vi "XAIOSCBG_v1.VI"(0 "BoardNum":u32, 1 "signal type":T2(ring)=enum."Sawtooth" caption="Signal Type", 2 "LowChan":i32, 3 "HighChan":i32=1, 5 "number of points":dbl=1024.0, 7 "amplitude (1.0)":dbl=10.0 caption="Amplitude (Volts)", 9 "offset (0.0)":dbl caption="Offset (Volts)", 11 "Range":i32(ring)=1 items=["Not Programmable"=0, "+- 20 V"=27, "+- 10 V"=1, "+- 5 V"=2, "+- 4 V"=28, "+- 2.5 V"=3, "+- 2 V"=29, "+- 1.67 V"=4, "+- 1.25 V"=5, "+- 1 V"=6, "+- .625 V"=7, "+- .5 V"=8, "+- .25 V"=30, "+- .2 V"=31, "+- .1 V"=9, "+- .05 V"=10, "+- .01 V"=11, "+- .005 V"=12, "0 - 10 V"=13, "0 - 5 V"=14, "0 - 4 V"=36, "0 - 2.5 V"=15, "0 - 2 V"=16, "0 - 1.67 V"=17, "0 - 1.25 V"=18, "0 - 1 V"=19, "0 - .5 V"=32, "0 - .25 V"=33, "0 - .2 V"=34, "0 - .1 V"=20, "0 - .02 V"=35, "0 - .01 V"=21, "4 - 20 mA"=22, "2 - 10 mA"=23, "1 - 5 mA"=24, ".5 - 2.5 mA"=25, "0 - 20 mA"=26], 12 "Rate":dbl=100.0, 13 "HighAOChan":i32, 14 "LowAOChan":i32) -> (4 "Output Array":dbl[][](array[numeric])=[[0.0, 0.006135884649154475, 0.012271538285719925, 0.01840672990580482, 0.024541228522912288, 0.030674803176636626, 0.03680722294135883, 0.04293825693494082, 0.049067674327418015, 0.05519524434968994, 0.06132073630220858, 0.06744391956366406, 0.07356456359966743, 0.07968243797143013, 0.0857973123444399, 0.09190895649713272, 0.0980171403295606, 0.10412163387205457, 0.11022220729388306, 0.11631863091190477, 0.1224106751992162, 0.12849811079379317, 0.1345807085071262, 0.14065823933284924, 0.14673047445536175, 0.15279718525844344, 0.15885814333386145, 0.16491312048996992, 0.17096188876030122, 0.17700422041214875, 0.18303988795514095, 0.18906866414980622, 0.19509032201612828, 0.2011046348420919, 0.20711137619221856, 0.21311031991609136, 0.2191012401568698, 0.22508391135979283, 0.2310581082806711, 0.2370236059943672, 0.2429801799032639, 0.24892760574572018, 0.25486565960451457, 0.2607941179152755, 0.26671275747489837, 0.272621355449949, 0.2785196893850531, 0.2844075372112718, 0.2902846772544624, 0.29615088824362384, 0.3020059493192281, 0.30784964004153487, 0.31368174039889146, 0.3195020308160157, 0.3253102921622629, 0.33110630575987643, 0.33688985339222005, 0.3426607173119944, 0.34841868024943456, 0.3541635254204904, 0.35989503653498817, 0.36561299780477385, 0.37131719395183754, 0.37700741021641826, 0.3826834323650898, 0.3883450466988263, 0.3939920400610481, 0.39962419984564684, 0.40524131400498986, 0.41084317105790397, 0.4164295600976372, 0.4220002707997997, 0.4275550934302821, 0.43309381885315196, 0.43861623853852766, 0.44412214457042926, 0.4496113296546066, 0.45508358712634384, 0.46053871095824, 0.4659764957679662, 0.47139673682599764, 0.47679923006332214, 0.4821837720791228, 0.48755016014843594, 0.49289819222978404, 0.49822766697278187, 0.5035383837257176, 0.508830142543107, 0.5141027441932218, 0.5193559901655896, 0.524589682678469, 0.5298036246862947, 0.5349976198870973, 0.5401714727298929, 0.5453249884220465, 0.5504579729366048, 0.5555702330196022, 0.560661576197336, 0.5657318107836132, 0.5707807458869673, 0.5758081914178453, 0.5808139580957645, 0.5857978574564389, 0.5907597018588743, 0.5956993044924334, 0.600616479383869, 0.6055110414043255, 0.6103828062763095, 0.6152315905806268, 0.6200572117632892, 0.6248594881423863, 0.629638238914927, 0.6343932841636455, 0.6391244448637757, 0.6438315428897915, 0.6485144010221124, 0.6531728429537768, 0.6578066932970786, 0.6624157775901718, 0.6669999223036375, 0.6715589548470184, 0.6760927035753159, 0.680600997795453, 0.6850836677727004, 0.6895405447370669, 0.693971460889654, 0.6983762494089728, 0.7027547444572253, 0.7071067811865476, 0.7114321957452164, 0.7157308252838187, 0.7200025079613817, 0.7242470829514669, 0.7284643904482252, 0.7326542716724128, 0.7368165688773699, 0.7409511253549591, 0.745057785441466, 0.7491363945234594, 0.7531867990436125, 0.7572088465064846, 0.7612023854842618, 0.765167265622459, 0.7691033376455796, 0.773010453362737, 0.7768884656732324, 0.7807372285720945, 0.7845565971555752, 0.7883464276266062, 0.7921065773002124, 0.7958369046088836, 0.799537269107905, 0.8032075314806449, 0.8068475535437992, 0.8104571982525948, 0.8140363297059484, 0.8175848131515837, 0.8211025149911046, 0.8245893027850253, 0.8280450452577558, 0.8314696123025452, 0.83486287498638, 0.8382247055548381, 0.8415549774368984, 0.8448535652497071, 0.8481203448032972, 0.8513551931052652, 0.8545579883654005, 0.8577286100002721, 0.8608669386377673, 0.8639728561215867, 0.8670462455156926, 0.8700869911087115, 0.8730949784182901, 0.8760700941954066, 0.8790122264286335, 0.881921264348355, 0.8847970984309378, 0.8876396204028539, 0.8904487232447579, 0.8932243011955153, 0.8959662497561851, 0.8986744656939538, 0.901348847046022, 0.9039892931234433, 0.9065957045149153, 0.9091679830905224, 0.9117060320054299, 0.9142097557035307, 0.9166790599210427, 0.9191138516900578, 0.9215140393420419, 0.9238795325112867, 0.9262102421383114, 0.9285060804732156, 0.9307669610789837, 0.9329927988347388, 0.9351835099389476, 0.937339011912575, 0.9394592236021899, 0.9415440651830208, 0.9435934581619604, 0.9456073253805213, 0.9475855910177411, 0.9495281805930367, 0.9514350209690083, 0.9533060403541939, 0.9551411683057707, 0.9569403357322088, 0.9587034748958716, 0.9604305194155658, 0.9621214042690416, 0.9637760657954398, 0.9653944416976894, 0.9669764710448521, 0.9685220942744173, 0.970031253194544, 0.9715038909862518, 0.9729399522055602, 0.9743393827855759, 0.9757021300385286, 0.9770281426577544, 0.9783173707196277, 0.9795697656854405, 0.9807852804032304, 0.9819638691095552, 0.9831054874312163, 0.984210092386929, 0.9852776423889412, 0.9863080972445987, 0.9873014181578584, 0.9882575677307495, 0.989176509964781, 0.9900582102622971, 0.99090263542778, 0.9917097536690995, 0.99247953459871, 0.9932119492347945, 0.9939069700023561, 0.9945645707342554, 0.9951847266721969, 0.9957674144676598, 0.996312612182778, 0.9968202992911657, 0.9972904566786902, 0.9977230666441916, 0.9981181129001492, 0.9984755805732948, 0.9987954562051724, 0.9990777277526454, 0.9993223845883495, 0.9995294175010931, 0.9996988186962042, 0.9998305817958234, 0.9999247018391445, 0.9999811752826011, 1.0, 0.9999811752826011, 0.9999247018391445, 0.9998305817958234, 0.9996988186962042, 0.9995294175010931, 0.9993223845883495, 0.9990777277526454, 0.9987954562051724, 0.9984755805732948, 0.9981181129001492, 0.9977230666441916, 0.9972904566786902, 0.9968202992911657, 0.996312612182778, 0.9957674144676598, 0.9951847266721969, 0.9945645707342554, 0.9939069700023561, 0.9932119492347945, 0.99247953459871, 0.9917097536690995, 0.99090263542778, 0.9900582102622971, 0.989176509964781, 0.9882575677307495, 0.9873014181578584, 0.9863080972445987, 0.9852776423889412, 0.984210092386929, 0.9831054874312163, 0.9819638691095552, 0.9807852804032304, 0.9795697656854405, 0.9783173707196277, 0.9770281426577544, 0.9757021300385286, 0.9743393827855759, 0.9729399522055602, 0.9715038909862518, 0.970031253194544, 0.9685220942744173, 0.9669764710448521, 0.9653944416976894, 0.9637760657954398, 0.9621214042690416, 0.9604305194155658, 0.9587034748958716, 0.9569403357322088, 0.9551411683057707, 0.9533060403541939, 0.9514350209690083, 0.9495281805930367, 0.9475855910177411, 0.9456073253805213, 0.9435934581619604, 0.9415440651830208, 0.9394592236021899, 0.937339011912575, 0.9351835099389476, 0.9329927988347388, 0.9307669610789837, 0.9285060804732156, 0.9262102421383114, 0.9238795325112867, 0.9215140393420419, 0.9191138516900578, 0.9166790599210427, 0.9142097557035307, 0.9117060320054299, 0.9091679830905224, 0.9065957045149153, 0.9039892931234433, 0.901348847046022, 0.8986744656939538, 0.8959662497561851, 0.8932243011955153, 0.8904487232447579, 0.8876396204028539, 0.8847970984309378, 0.881921264348355, 0.8790122264286335, 0.8760700941954066, 0.8730949784182901, 0.8700869911087115, 0.8670462455156926, 0.8639728561215867, 0.8608669386377673, 0.8577286100002721, 0.8545579883654005, 0.8513551931052652, 0.8481203448032972, 0.8448535652497071, 0.8415549774368984, 0.8382247055548381, 0.83486287498638, 0.8314696123025452, 0.8280450452577558, 0.8245893027850253, 0.8211025149911046, 0.8175848131515837, 0.8140363297059484, 0.8104571982525948, 0.8068475535437992, 0.8032075314806449, 0.799537269107905, 0.7958369046088836, 0.7921065773002124, 0.7883464276266062, 0.7845565971555752, 0.7807372285720945, 0.7768884656732324, 0.773010453362737, 0.7691033376455796, 0.765167265622459, 0.7612023854842618, 0.7572088465064846, 0.7531867990436125, 0.7491363945234594, 0.745057785441466, 0.7409511253549591, 0.7368165688773699, 0.7326542716724128, 0.7284643904482252, 0.7242470829514669, 0.7200025079613817, 0.7157308252838187, 0.7114321957452164, 0.7071067811865476, 0.7027547444572253, 0.6983762494089728, 0.693971460889654, 0.6895405447370669, 0.6850836677727004, 0.680600997795453, 0.6760927035753159, 0.6715589548470184, 0.6669999223036375, 0.6624157775901718, 0.6578066932970786, 0.6531728429537768, 0.6485144010221124, 0.6438315428897915, 0.6391244448637757, 0.6343932841636455, 0.629638238914927, 0.6248594881423863, 0.6200572117632892, 0.6152315905806268, 0.6103828062763095, 0.6055110414043255, 0.600616479383869, 0.5956993044924334, 0.5907597018588743, 0.5857978574564389, 0.5808139580957645, 0.5758081914178453, 0.5707807458869673, 0.5657318107836132, 0.560661576197336, 0.5555702330196022, 0.5504579729366048, 0.5453249884220465, 0.5401714727298929, 0.5349976198870973, 0.5298036246862947, 0.524589682678469, 0.5193559901655896, 0.5141027441932218, 0.508830142543107, 0.5035383837257176, 0.49822766697278187, 0.49289819222978404, 0.48755016014843594, 0.4821837720791228, 0.47679923006332214, 0.47139673682599764, 0.4659764957679662, 0.46053871095824, 0.45508358712634384, 0.4496113296546066, 0.44412214457042926, 0.43861623853852766, 0.43309381885315196, 0.4275550934302821, 0.4220002707997997, 0.4164295600976372, 0.41084317105790397, 0.40524131400498986, 0.39962419984564684, 0.3939920400610481, 0.3883450466988263, 0.3826834323650898, 0.37700741021641826, 0.37131719395183754, 0.36561299780477385, 0.35989503653498817, 0.3541635254204904, 0.34841868024943456, 0.3426607173119944, 0.33688985339222005, 0.33110630575987643, 0.3253102921622629, 0.3195020308160157, 0.31368174039889146, 0.30784964004153487, 0.3020059493192281, 0.29615088824362384, 0.2902846772544624, 0.2844075372112718, 0.2785196893850531, 0.272621355449949, 0.26671275747489837, 0.2607941179152755, 0.25486565960451457, 0.24892760574572018, 0.2429801799032639, 0.2370236059943672, 0.2310581082806711, 0.22508391135979283, 0.2191012401568698, 0.21311031991609136, 0.20711137619221856, 0.2011046348420919, 0.19509032201612828, 0.18906866414980622, 0.18303988795514095, 0.17700422041214875, 0.17096188876030122, 0.16491312048996992, 0.15885814333386145, 0.15279718525844344, 0.14673047445536175, 0.14065823933284924, 0.1345807085071262, 0.12849811079379317, 0.1224106751992162, 0.11631863091190477, 0.11022220729388306, 0.10412163387205457, 0.0980171403295606, 0.09190895649713272, 0.0857973123444399, 0.07968243797143013, 0.07356456359966743, 0.06744391956366405, 0.06132073630220858, 0.05519524434968994, 0.049067674327418015, 0.04293825693494082, 0.03680722294135883, 0.030674803176636626, 0.024541228522912288, 0.01840672990580482, 0.012271538285719925, 0.006135884649154475, -5.421010862427522e-20, -0.006135884649154475, -0.012271538285719925, -0.01840672990580482, -0.024541228522912288, -0.030674803176636626, -0.03680722294135883, -0.04293825693494082, -0.049067674327418015, -0.05519524434968994, -0.06132073630220858, -0.06744391956366406, -0.07356456359966743, -0.07968243797143013, -0.0857973123444399, -0.09190895649713272, -0.0980171403295606, -0.10412163387205457, -0.11022220729388306, -0.11631863091190477, -0.1224106751992162, -0.12849811079379317, -0.1345807085071262, -0.14065823933284924, -0.14673047445536175, -0.15279718525844344, -0.15885814333386145, -0.16491312048996992, -0.17096188876030122, -0.17700422041214875, -0.18303988795514095, -0.18906866414980622, -0.19509032201612828, -0.2011046348420919, -0.20711137619221856, -0.21311031991609136, -0.2191012401568698, -0.22508391135979283, -0.2310581082806711, -0.2370236059943672, -0.2429801799032639, -0.24892760574572018, -0.25486565960451457, -0.2607941179152755, -0.26671275747489837, -0.272621355449949, -0.2785196893850531, -0.2844075372112718, -0.2902846772544624, -0.29615088824362384, -0.3020059493192281, -0.30784964004153487, -0.31368174039889146, -0.3195020308160157, -0.3253102921622629, -0.33110630575987643, -0.33688985339222005, -0.3426607173119944, -0.34841868024943456, -0.3541635254204904, -0.35989503653498817, -0.36561299780477385, -0.37131719395183754, -0.37700741021641826, -0.3826834323650898, -0.3883450466988263, -0.3939920400610481, -0.39962419984564684, -0.40524131400498986, -0.41084317105790397, -0.4164295600976372, -0.4220002707997997, -0.4275550934302821, -0.43309381885315196, -0.43861623853852766, -0.44412214457042926, -0.4496113296546066, -0.45508358712634384, -0.46053871095824, -0.4659764957679662, -0.47139673682599764, -0.47679923006332214, -0.4821837720791228, -0.48755016014843594, -0.49289819222978404, -0.49822766697278187, -0.5035383837257176, -0.508830142543107, -0.5141027441932218, -0.5193559901655896, -0.524589682678469, -0.5298036246862947, -0.5349976198870973, -0.5401714727298929, -0.5453249884220465, -0.5504579729366048, -0.5555702330196022, -0.560661576197336, -0.5657318107836132, -0.5707807458869673, -0.5758081914178453, -0.5808139580957645, -0.5857978574564389, -0.5907597018588743, -0.5956993044924334, -0.600616479383869, -0.6055110414043255, -0.6103828062763095, -0.6152315905806268, -0.6200572117632892, -0.6248594881423863, -0.629638238914927, -0.6343932841636455, -0.6391244448637757, -0.6438315428897915, -0.6485144010221124, -0.6531728429537768, -0.6578066932970786, -0.6624157775901718, -0.6669999223036375, -0.6715589548470184, -0.6760927035753159, -0.680600997795453, -0.6850836677727004, -0.6895405447370669, -0.693971460889654, -0.6983762494089728, -0.7027547444572253, -0.7071067811865476, -0.7114321957452164, -0.7157308252838187, -0.7200025079613817, -0.7242470829514669, -0.7284643904482252, -0.7326542716724128, -0.7368165688773699, -0.7409511253549591, -0.745057785441466, -0.7491363945234594, -0.7531867990436125, -0.7572088465064846, -0.7612023854842618, -0.765167265622459, -0.7691033376455796, -0.773010453362737, -0.7768884656732324, -0.7807372285720945, -0.7845565971555752, -0.7883464276266062, -0.7921065773002124, -0.7958369046088836, -0.799537269107905, -0.8032075314806449, -0.8068475535437992, -0.8104571982525948, -0.8140363297059484, -0.8175848131515837, -0.8211025149911046, -0.8245893027850253, -0.8280450452577558, -0.8314696123025452, -0.83486287498638, -0.8382247055548381, -0.8415549774368984, -0.8448535652497071, -0.8481203448032972, -0.8513551931052652, -0.8545579883654005, -0.8577286100002721, -0.8608669386377673, -0.8639728561215867, -0.8670462455156926, -0.8700869911087115, -0.8730949784182901, -0.8760700941954066, -0.8790122264286335, -0.881921264348355, -0.8847970984309378, -0.8876396204028539, -0.8904487232447579, -0.8932243011955153, -0.8959662497561851, -0.8986744656939538, -0.901348847046022, -0.9039892931234433, -0.9065957045149153, -0.9091679830905224, -0.9117060320054299, -0.9142097557035307, -0.9166790599210427, -0.9191138516900578, -0.9215140393420419, -0.9238795325112867, -0.9262102421383114, -0.9285060804732156, -0.9307669610789837, -0.9329927988347388, -0.9351835099389476, -0.937339011912575, -0.9394592236021899, -0.9415440651830208, -0.9435934581619604, -0.9456073253805213, -0.9475855910177411, -0.9495281805930367, -0.9514350209690083, -0.9533060403541939, -0.9551411683057707, -0.9569403357322088, -0.9587034748958716, -0.9604305194155658, -0.9621214042690416, -0.9637760657954398, -0.9653944416976894, -0.9669764710448521, -0.9685220942744173, -0.970031253194544, -0.9715038909862518, -0.9729399522055602, -0.9743393827855759, -0.9757021300385286, -0.9770281426577544, -0.9783173707196277, -0.9795697656854405, -0.9807852804032304, -0.9819638691095552, -0.9831054874312163, -0.984210092386929, -0.9852776423889412, -0.9863080972445987, -0.9873014181578584, -0.9882575677307495, -0.989176509964781, -0.9900582102622971, -0.99090263542778, -0.9917097536690995, -0.99247953459871, -0.9932119492347945, -0.9939069700023561, -0.9945645707342554, -0.9951847266721969, -0.9957674144676598, -0.996312612182778, -0.9968202992911657, -0.9972904566786902, -0.9977230666441916, -0.9981181129001492, -0.9984755805732948, -0.9987954562051724, -0.9990777277526454, -0.9993223845883495, -0.9995294175010931, -0.9996988186962042, -0.9998305817958234, -0.9999247018391445, -0.9999811752826011, -1.0, -0.9999811752826011, -0.9999247018391445, -0.9998305817958234, -0.9996988186962042, -0.9995294175010931, -0.9993223845883495, -0.9990777277526454, -0.9987954562051724, -0.9984755805732948, -0.9981181129001492, -0.9977230666441916, -0.9972904566786902, -0.9968202992911657, -0.996312612182778, -0.9957674144676598, -0.9951847266721969, -0.9945645707342554, -0.9939069700023561, -0.9932119492347945, -0.99247953459871, -0.9917097536690995, -0.99090263542778, -0.9900582102622971, -0.989176509964781, -0.9882575677307495, -0.9873014181578584, -0.9863080972445987, -0.9852776423889412, -0.984210092386929, -0.9831054874312163, -0.9819638691095552, -0.9807852804032304, -0.9795697656854405, -0.9783173707196277, -0.9770281426577544, -0.9757021300385286, -0.9743393827855759, -0.9729399522055602, -0.9715038909862518, -0.970031253194544, -0.9685220942744173, -0.9669764710448521, -0.9653944416976894, -0.9637760657954398, -0.9621214042690416, -0.9604305194155658, -0.9587034748958716, -0.9569403357322088, -0.9551411683057707, -0.9533060403541939, -0.9514350209690083, -0.9495281805930367, -0.9475855910177411, -0.9456073253805213, -0.9435934581619604, -0.9415440651830208, -0.9394592236021899, -0.937339011912575, -0.9351835099389476, -0.9329927988347388, -0.9307669610789837, -0.9285060804732156, -0.9262102421383114, -0.9238795325112867, -0.9215140393420419, -0.9191138516900578, -0.9166790599210427, -0.9142097557035307, -0.9117060320054299, -0.9091679830905224, -0.9065957045149153, -0.9039892931234433, -0.901348847046022, -0.8986744656939538, -0.8959662497561851, -0.8932243011955153, -0.8904487232447579, -0.8876396204028539, -0.8847970984309378, -0.881921264348355, -0.8790122264286335, -0.8760700941954066, -0.8730949784182901, -0.8700869911087115, -0.8670462455156926, -0.8639728561215867, -0.8608669386377673, -0.8577286100002721, -0.8545579883654005, -0.8513551931052652, -0.8481203448032972, -0.8448535652497071, -0.8415549774368984, -0.8382247055548381, -0.83486287498638, -0.8314696123025452, -0.8280450452577558, -0.8245893027850253, -0.8211025149911046, -0.8175848131515837, -0.8140363297059484, -0.8104571982525948, -0.8068475535437992, -0.8032075314806449, -0.799537269107905, -0.7958369046088836, -0.7921065773002124, -0.7883464276266062, -0.7845565971555752, -0.7807372285720945, -0.7768884656732324, -0.773010453362737, -0.7691033376455796, -0.765167265622459, -0.7612023854842618, -0.7572088465064846, -0.7531867990436125, -0.7491363945234594, -0.745057785441466, -0.7409511253549591, -0.7368165688773699, -0.7326542716724128, -0.7284643904482252, -0.7242470829514669, -0.7200025079613817, -0.7157308252838187, -0.7114321957452164, -0.7071067811865476, -0.7027547444572253, -0.6983762494089728, -0.693971460889654, -0.6895405447370669, -0.6850836677727004, -0.680600997795453, -0.6760927035753159, -0.6715589548470184, -0.6669999223036375, -0.6624157775901718, -0.6578066932970786, -0.6531728429537768, -0.6485144010221124, -0.6438315428897915, -0.6391244448637757, -0.6343932841636455, -0.629638238914927, -0.6248594881423863, -0.6200572117632892, -0.6152315905806268, -0.6103828062763095, -0.6055110414043255, -0.600616479383869, -0.5956993044924334, -0.5907597018588743, -0.5857978574564389, -0.5808139580957645, -0.5758081914178453, -0.5707807458869673, -0.5657318107836132, -0.560661576197336, -0.5555702330196022, -0.5504579729366048, -0.5453249884220465, -0.5401714727298929, -0.5349976198870973, -0.5298036246862947, -0.524589682678469, -0.5193559901655896, -0.5141027441932218, -0.508830142543107, -0.5035383837257176, -0.49822766697278187, -0.49289819222978404, -0.48755016014843594, -0.4821837720791228, -0.47679923006332214, -0.47139673682599764, -0.4659764957679662, -0.46053871095824, -0.45508358712634384, -0.4496113296546066, -0.44412214457042926, -0.43861623853852766, -0.43309381885315196, -0.4275550934302821, -0.4220002707997997, -0.4164295600976372, -0.41084317105790397, -0.40524131400498986, -0.39962419984564684, -0.3939920400610481, -0.3883450466988263, -0.3826834323650898, -0.37700741021641826, -0.37131719395183754, -0.36561299780477385, -0.35989503653498817, -0.3541635254204904, -0.34841868024943456, -0.3426607173119944, -0.33688985339222005, -0.33110630575987643, -0.3253102921622629, -0.3195020308160157, -0.31368174039889146, -0.30784964004153487, -0.3020059493192281, -0.29615088824362384, -0.2902846772544624, -0.2844075372112718, -0.2785196893850531, -0.272621355449949, -0.26671275747489837, -0.2607941179152755, -0.25486565960451457, -0.24892760574572018, -0.2429801799032639, -0.2370236059943672, -0.2310581082806711, -0.22508391135979283, -0.2191012401568698, -0.21311031991609136, -0.20711137619221856, -0.2011046348420919, -0.19509032201612828, -0.18906866414980622, -0.18303988795514095, -0.17700422041214875, -0.17096188876030122, -0.16491312048996992, -0.15885814333386145, -0.15279718525844344, -0.14673047445536175, -0.14065823933284924, -0.1345807085071262, -0.12849811079379317, -0.1224106751992162, -0.11631863091190477, -0.11022220729388306, -0.10412163387205457, -0.0980171403295606, -0.09190895649713272, -0.0857973123444399, -0.07968243797143013, -0.07356456359966743, -0.06744391956366405, -0.06132073630220858, -0.05519524434968994, -0.049067674327418015, -0.04293825693494082, -0.03680722294135883, -0.030674803176636626, -0.024541228522912288, -0.01840672990580482, -0.012271538285719925, -0.006135884649154475]] min=0.0 max=0.0 format="%.2f", 6 "AIn-ErrCode":i32, 8 "OutContext":T1={"IntnlBoardNum"=0, "Data"=[0, 0, 0, 0, 0, 0, 0, 0, 0, 0, 0, 0, 0, 0, 0, 0, 0, 0, 0, 0, 0, 0, 0, 0, 0, 0, 0, 0, 0, 0, 0, 0, 0, 0, 0, 0, 0, 0, 0, 0, 0, 0, 0, 0, 0, 0, 0, 0, 0, 0, 0, 0, 0, 0, 0, 0, 0, 0, 0, 0, 0, 0, 0, 0, 0, 0, 0, 0, 0, 0, 0, 0, 0, 0, 0, 0, 0, 0, 0, 0, 0, 0, 0, 0, 0, 0, 0, 0, 0, 0, 0, 0, 0, 0, 0, 0, 0, 0, 0, 0, 0, 0, 0, 0, 0, 0, 0, 0, 0, 0, 0, 0, 0, 0, 0, 0, 0, 0, 0, 0, 0, 0, 0, 0, 0, 0, 0, 0, 0, 0, 0, 0, 0, 0, 0, 0, 0, 0, 0, 0, 0, 0, 0, 0, 0, 0, 0, 0, 0, 0, 0, 0, 0, 0, 0, 0, 0, 0, 0, 0, 0, 0, 0, 0, 0, 0, 0, 0, 0, 0, 0, 0, 0, 0, 0, 0, 0, 0, 0, 0, 0, 0, 0, 0, 0, 0, 0, 0, 0, 0, 0, 0, 0, 0, 0, 0, 0, 0, 0, 0, 0, 0, 0, 0, 0, 0, 0, 0, 0, 0, 0, 0, 0, 0, 0, 0, 0, 0, 0, 0, 0, 0, 0, 0, 0, 0, 0, 0, 0, 0, 0, 0, 0, 0, 0, 0, 0, 0, 0, 0, 0, 0, 0, 0, 0, 0, 0, 0, 0, 0, 0, 0, 0, 0, 0, 0, 0, 0, 0, 0, 0, 0, 0, 0, 0, 0, 0, 0, 0, 0, 0, 0, 0, 0, 0, 0, 0, 0, 0, 0, 0, 0, 0, 0, 0, 0, 0, 0, 0, 0, 0, 0, 0, 0, 0, 0, 0, 0, 0, 0, 0, 0, 0, 0, 0, 0, 0, 0, 0, 0, 0, 0, 0, 0, 0, 0, 0, 0, 0, 0, 0, 0, 0, 0, 0, 0, 0, 0, 0, 0, 0, 0, 0, 0, 0, 0, 0, 0, 0, 0, 0, 0, 0, 0, 0, 0, 0, 0, 0, 0, 0, 0, 0, 0, 0, 0, 0, 0, 0, 0, 0, 0, 0, 0, 0, 0, 0, 0, 0, 0, 0, 0, 0, 0, 0, 0, 0, 0, 0, 0, 0, 0, 0, 0, 0, 0, 0, 0, 0, 0, 0, 0, 0, 0, 0, 0, 0, 0, 0, 0, 0, 0, 0, 0, 0, 0, 0, 0, 0, 0, 0, 0, 0, 0, 0, 0, 0, 0, 0, 0, 0, 0, 0, 0, 0, 0, 0, 0, 0, 0, 0, 0, 0, 0, 0, 0, 0, 0, 0, 0, 0, 0, 0, 0, 0, 0, 0, 0, 0, 0, 0, 0, 0, 0, 0, 0, 0, 0, 0, 0, 0, 0, 0, 0, 0, 0, 0, 0, 0, 0, 0, 0, 0, 0, 0, 0, 0, 0, 0, 0, 0, 0, 0, 0, 0, 0, 0, 0, 0, 0, 0, 0, 0, 0, 0, 0, 0, 0, 0, 0, 0, 0, 0, 0, 0, 0, 0, 0, 0, 0, 0, 0, 0, 0, 0, 0, 0, 0, 0, 0, 0, 0, 0, 0, 0, 0, 0, 0, 0, 0, 0, 0, 0, 0, 0, 0, 0, 0, 0, 0, 0, 0, 0, 0, 0, 0, 0, 0, 0, 0, 0, 0, 0, 0, 0, 0, 0, 0, 0, 0, 0, 0, 0, 0, 0, 0, 0, 0, 0, 0, 0, 0, 0, 0, 0, 0, 0, 0, 0, 0, 0, 0, 0, 0, 0, 0, 0, 0, 0, 0, 0, 0, 0, 0, 0, 0, 0, 0, 0, 0, 0, 0, 0, 0, 0, 0, 0, 0, 0, 0, 0, 0, 0, 0, 0, 0, 0, 0, 0, 0, 0, 0, 0, 0, 0, 0, 0, 0, 0, 0, 0, 0, 0, 0, 0, 0, 0, 0, 0, 0, 0, 0, 0, 0, 0, 0, 0, 0, 0, 0, 0, 0, 0, 0, 0, 0, 0, 0, 0, 0, 0, 0, 0, 0, 0, 0, 0, 0, 0, 0, 0, 0, 0, 0, 0, 0, 0, 0, 0, 0, 0, 0, 0, 0, 0, 0, 0, 0, 0, 0, 0, 0, 0, 0, 0, 0, 0, 0, 0, 0, 0, 0, 0, 0, 0, 0, 0, 0, 0, 0, 0, 0, 0, 0, 0, 0, 0, 0, 0, 0, 0, 0, 0, 0, 0, 0, 0, 0, 0, 0, 0, 0, 0, 0, 0, 0, 0, 0, 0, 0, 0, 0, 0, 0, 0, 0, 0, 0, 0, 0, 0, 0, 0, 0, 0, 0, 0, 0, 0, 0, 0, 0, 0, 0, 0, 0, 0, 0, 0, 0, 0, 0, 0, 0, 0, 0, 0, 0, 0, 0, 0, 0, 0, 0, 0, 0, 0, 0, 0, 0, 0, 0, 0, 0, 0, 0, 0, 0, 0, 0, 0, 0, 0, 0, 0, 0, 0, 0, 0, 0, 0, 0, 0, 0, 0, 0, 0, 0, 0, 0, 0, 0, 0, 0, 0, 0, 0, 0, 0, 0, 0, 0, 0, 0, 0, 0, 0, 0, 0, 0, 0, 0, 0, 0, 0, 0, 0, 0, 0, 0, 0, 0, 0, 0, 0, 0, 0, 0, 0, 0, 0, 0, 0, 0, 0, 0, 0, 0, 0, 0, 0, 0, 0, 0, 0, 0, 0, 0, 0, 0, 0, 0, 0, 0, 0, 0, 0, 0, 0, 0, 0, 0, 0, 0, 0, 0, 0, 0, 0, 0, 0, 0, 0, 0, 0, 0, 0, 0, 0, 0, 0, 0, 0, 0, 0, 0, 0, 0, 0, 0, 0, 0, 0, 0, 0, 0, 0, 0, 0, 0, 0, 0, 0, 0, 0, 0, 0, 0, 0, 0, 0, 0, 0, 0, 0, 0, 0, 0, 0, 0, 0, 0, 0, 0, 0, 0, 0, 0, 0, 0, 0, 0, 0, 0, 0, 0, 0, 0, 0, 0, 0, 0, 0, 0, 0, 0, 0, 0, 0, 0, 0, 0, 0, 0, 0, 0, 0, 0, 0, 0, 0, 0, 0, 0, 0, 0, 0, 0, 0, 0, 0, 0, 0, 0, 0, 0, 0, 0, 0, 0, 0, 0, 0, 0, 0, 0, 0, 0, 0, 0, 0, 0, 0, 0], "Size"=0, "IntnlStatus"=0, "IntnlErrCode"=93, "Alias16"=0, "Reserved"=0}, 10 "AOut-ErrCode":i32, 15 "InContext":T1={"IntnlBoardNum"=0, "Data"=[0, 0, 0, 0, 0, 0, 0, 0, 0, 0, 0, 0, 0, 0, 0, 0, 0, 0, 0, 0, 0, 0, 0, 0, 0, 0, 0, 0, 0, 0, 0, 0, 0, 0, 0, 0, 0, 0, 0, 0, 0, 0, 0, 0, 0, 0, 0, 0, 0, 0, 0, 0, 0, 0, 0, 0, 0, 0, 0, 0, 0, 0, 0, 0, 0, 0, 0, 0, 0, 0, 0, 0, 0, 0, 0, 0, 0, 0, 0, 0, 0, 0, 0, 0, 0, 0, 0, 0, 0, 0, 0, 0, 0, 0, 0, 0, 0, 0, 0, 0, 0, 0, 0, 0, 0, 0, 0, 0, 0, 0, 0, 0, 0, 0, 0, 0, 0, 0, 0, 0, 0, 0, 0, 0, 0, 0, 0, 0, 0, 0, 0, 0, 0, 0, 0, 0, 0, 0, 0, 0, 0, 0, 0, 0, 0, 0, 0, 0, 0, 0, 0, 0, 0, 0, 0, 0, 0, 0, 0, 0, 0, 0, 0, 0, 0, 0, 0, 0, 0, 0, 0, 0, 0, 0, 0, 0, 0, 0, 0, 0, 0, 0, 0, 0, 0, 0, 0, 0, 0, 0, 0, 0, 0, 0, 0, 0, 0, 0, 0, 0, 0, 0, 0, 0, 0, 0, 0, 0, 0, 0, 0, 0, 0, 0, 0, 0, 0, 0, 0, 0, 0, 0, 0, 0, 0, 0, 0, 0, 0, 0, 0, 0, 0, 0, 0, 0, 0, 0, 0, 0, 0, 0, 0, 0, 0, 0, 0, 0, 0, 0, 0, 0, 0, 0, 0, 0, 0, 0, 0, 0, 0, 0, 0, 0, 0, 0, 0, 0, 0, 0, 0, 0, 0, 0, 0, 0, 0, 0, 0, 0, 0, 0, 0, 0, 0, 0, 0, 0, 0, 0, 0, 0, 0, 0, 0, 0, 0, 0, 0, 0, 0, 0, 0, 0, 0, 0, 0, 0, 0, 0, 0, 0, 0, 0, 0, 0, 0, 0, 0, 0, 0, 0, 0, 0, 0, 0, 0, 0, 0, 0, 0, 0, 0, 0, 0, 0, 0, 0, 0, 0, 0, 0, 0, 0, 0, 0, 0, 0, 0, 0, 0, 0, 0, 0, 0, 0, 0, 0, 0, 0, 0, 0, 0, 0, 0, 0, 0, 0, 0, 0, 0, 0, 0, 0, 0, 0, 0, 0, 0, 0, 0, 0, 0, 0, 0, 0, 0, 0, 0, 0, 0, 0, 0, 0, 0, 0, 0, 0, 0, 0, 0, 0, 0, 0, 0, 0, 0, 0, 0, 0, 0, 0, 0, 0, 0, 0, 0, 0, 0, 0, 0, 0, 0, 0, 0, 0, 0, 0, 0, 0, 0, 0, 0, 0, 0, 0, 0, 0, 0, 0, 0, 0, 0, 0, 0, 0, 0, 0, 0, 0, 0, 0, 0, 0, 0, 0, 0, 0, 0, 0, 0, 0, 0, 0, 0, 0, 0, 0, 0, 0, 0, 0, 0, 0, 0, 0, 0, 0, 0, 0, 0, 0, 0, 0, 0, 0, 0, 0, 0, 0, 0, 0, 0, 0, 0, 0, 0, 0, 0, 0, 0, 0, 0, 0, 0, 0, 0, 0, 0, 0, 0, 0, 0, 0, 0, 0, 0, 0, 0, 0, 0, 0, 0, 0, 0, 0, 0, 0, 0, 0, 0, 0, 0, 0, 0, 0, 0, 0, 0, 0, 0, 0, 0, 0, 0, 0, 0, 0, 0, 0, 0, 0, 0, 0, 0, 0, 0, 0, 0, 0, 0, 0, 0, 0, 0, 0, 0, 0, 0, 0, 0, 0, 0, 0, 0, 0, 0, 0, 0, 0, 0, 0, 0, 0, 0, 0, 0, 0, 0, 0, 0, 0, 0, 0, 0, 0, 0, 0, 0, 0, 0, 0, 0, 0, 0, 0, 0, 0, 0, 0, 0, 0, 0, 0, 0, 0, 0, 0, 0, 0, 0, 0, 0, 0, 0, 0, 0, 0, 0, 0, 0, 0, 0, 0, 0, 0, 0, 0, 0, 0, 0, 0, 0, 0, 0, 0, 0, 0, 0, 0, 0, 0, 0, 0, 0, 0, 0, 0, 0, 0, 0, 0, 0, 0, 0, 0, 0, 0, 0, 0, 0, 0, 0, 0, 0, 0, 0, 0, 0, 0, 0, 0, 0, 0, 0, 0, 0, 0, 0, 0, 0, 0, 0, 0, 0, 0, 0, 0, 0, 0, 0, 0, 0, 0, 0, 0, 0, 0, 0, 0, 0, 0, 0, 0, 0, 0, 0, 0, 0, 0, 0, 0, 0, 0, 0, 0, 0, 0, 0, 0, 0, 0, 0, 0, 0, 0, 0, 0, 0, 0, 0, 0, 0, 0, 0, 0, 0, 0, 0, 0, 0, 0, 0, 0, 0, 0, 0, 0, 0, 0, 0, 0, 0, 0, 0, 0, 0, 0, 0, 0, 0, 0, 0, 0, 0, 0, 0, 0, 0, 0, 0, 0, 0, 0, 0, 0, 0, 0, 0, 0, 0, 0, 0, 0, 0, 0, 0, 0, 0, 0, 0, 0, 0, 0, 0, 0, 0, 0, 0, 0, 0, 0, 0, 0, 0, 0, 0, 0, 0, 0, 0, 0, 0, 0, 0, 0, 0, 0, 0, 0, 0, 0, 0, 0, 0, 0, 0, 0, 0, 0, 0, 0, 0, 0, 0, 0, 0, 0, 0, 0, 0, 0, 0, 0, 0, 0, 0, 0, 0, 0, 0, 0, 0, 0, 0, 0, 0, 0, 0, 0, 0, 0, 0, 0, 0, 0, 0, 0, 0, 0, 0, 0, 0, 0, 0, 0, 0, 0, 0, 0, 0, 0, 0, 0, 0, 0, 0, 0, 0, 0, 0, 0, 0, 0, 0, 0, 0, 0, 0, 0, 0, 0, 0, 0, 0, 0, 0, 0, 0, 0, 0, 0, 0, 0, 0, 0, 0, 0, 0, 0, 0, 0, 0, 0, 0, 0, 0, 0, 0, 0, 0, 0, 0, 0, 0, 0, 0, 0, 0, 0, 0, 0, 0, 0, 0, 0, 0, 0, 0, 0, 0, 0, 0, 0, 0, 0, 0, 0, 0, 0, 0, 0, 0, 0, 0, 0, 0, 0, 0, 0, 0, 0, 0, 0, 0, 0, 0, 0, 0, 0, 0, 0, 0, 0, 0, 0, 0, 0, 0, 0, 0, 0, 0, 0, 0, 0, 0, 0, 0, 0, 0, 0, 0, 0, 0, 0, 0, 0, 0, 0, 0, 0, 0, 0, 0, 0, 0, 0, 0, 0, 0, 0, 0, 0, 0, 0, 0, 0, 0, 0, 0, 0, 0, 0, 0, 0, 0, 0, 0, 0, 0, 0, 0, 0, 0, 0, 0, 0, 0, 0, 0, 0, 0, 0, 0, 0, 0, 0, 0, 0, 0, 0, 0, 0, 0, 0, 0, 0, 0, 0, 0, 0, 0, 0, 0, 0, 0, 0, 0, 0, 0, 0, 0, 0, 0, 0, 0, 0, 0, 0, 0, 0, 0, 0, 0, 0, 0, 0, 0, 0, 0, 0, 0, 0, 0, 0, 0, 0, 0, 0, 0, 0, 0, 0, 0, 0, 0, 0, 0, 0, 0, 0, 0, 0, 0, 0, 0, 0, 0, 0, 0, 0, 0, 0, 0, 0, 0, 0, 0, 0, 0, 0, 0, 0, 0, 0, 0, 0, 0, 0, 0, 0, 0, 0, 0, 0, 0, 0, 0, 0, 0, 0, 0, 0, 0, 0, 0, 0, 0, 0, 0, 0, 0, 0, 0, 0, 0, 0, 0, 0, 0, 0, 0, 0, 0, 0, 0, 0, 0, 0, 0, 0, 0, 0, 0, 0, 0, 0, 0, 0, 0, 0, 0, 0, 0, 0, 0, 0, 0, 0, 0, 0, 0, 0, 0, 0, 0, 0, 0, 0, 0, 0, 0, 0, 0, 0, 0, 0, 0, 0, 0, 0, 0, 0, 0, 0, 0, 0, 0, 0, 0, 0, 0, 0, 0, 0, 0, 0, 0, 0, 0, 0, 0, 0, 0, 0, 0, 0, 0, 0, 0, 0, 0, 0, 0, 0, 0, 0, 0, 0, 0, 0, 0, 0, 0, 0, 0, 0, 0, 0, 0, 0, 0, 0, 0, 0, 0, 0, 0, 0, 0, 0, 0, 0, 0, 0, 0, 0, 0, 0, 0, 0, 0, 0, 0, 0, 0, 0, 0, 0, 0, 0, 0, 0, 0, 0, 0, 0, 0, 0, 0, 0, 0, 0, 0, 0, 0, 0, 0, 0, 0, 0, 0, 0, 0, 0, 0, 0, 0, 0, 0, 0, 0, 0, 0, 0, 0, 0, 0, 0, 0, 0, 0, 0, 0, 0, 0, 0, 0, 0, 0, 0, 0, 0, 0, 0, 0, 0, 0, 0, 0, 0, 0, 0, 0, 0, 0, 0, 0, 0, 0, 0, 0, 0, 0, 0, 0, 0, 0, 0, 0, 0, 0, 0, 0, 0, 0, 0, 0, 0, 0, 0, 0, 0, 0, 0, 0, 0, 0, 0, 0, 0, 0, 0, 0, 0, 0, 0, 0, 0, 0, 0, 0, 0, 0, 0, 0, 0, 0, 0, 0, 0, 0, 0, 0, 0, 0, 0, 0, 0, 0, 0, 0, 0, 0, 0, 0, 0, 0, 0, 0, 0, 0, 0, 0, 0, 0, 0, 0, 0, 0, 0, 0, 0, 0, 0, 0, 0, 0, 0, 0, 0, 0, 0, 0, 0, 0, 0, 0, 0, 0, 0, 0, 0, 0, 0, 0, 0, 0, 0, 0, 0, 0, 0, 0, 0, 0, 0, 0, 0, 0, 0, 0, 0, 0, 0, 0, 0, 0, 0, 0, 0, 0, 0, 0, 0, 0, 0, 0, 0, 0, 0, 0, 0, 0, 0, 0, 0, 0, 0, 0, 0, 0, 0, 0, 0, 0, 0, 0, 0, 0, 0, 0, 0, 0, 0, 0, 0, 0, 0, 0, 0, 0, 0, 0, 0, 0, 0, 0, 0, 0, 0, 0, 0, 0, 0, 0, 0, 0, 0, 0, 0, 0, 0, 0, 0, 0, 0, 0, 0, 0, 0, 0, 0, 0, 0, 0, 0, 0, 0, 0, 0, 0, 0, 0, 0, 0, 0, 0, 0, 0, 0, 0, 0, 0, 0, 0, 0, 0, 0, 0, 0, 0, 0, 0, 0, 0, 0, 0, 0, 0, 0, 0, 0, 0, 0, 0, 0, 0, 0, 0, 0, 0, 0, 0, 0, 0, 0, 0, 0, 0, 0, 0, 0, 0, 0, 0, 0, 0, 0, 0, 0, 0, 0, 0, 0, 0, 0, 0, 0, 0, 0, 0, 0, 0, 0, 0, 0, 0, 0, 0, 0, 0, 0, 0, 0, 0, 0, 0, 0, 0, 0, 0, 0, 0, 0, 0, 0, 0, 0, 0, 0, 0, 0, 0, 0, 0, 0, 0, 0, 0, 0, 0, 0, 0, 0, 0, 0, 0, 0, 0, 0, 0, 0, 0, 0, 0, 0, 0, 0, 0, 0, 0, 0, 0, 0, 0, 0, 0, 0, 0, 0, 0, 0, 0, 0, 0, 0, 0, 0, 0, 0, 0, 0, 0, 0, 0, 0, 0, 0, 0, 0, 0, 0, 0, 0, 0, 0, 0, 0, 0, 0, 0, 0, 0, 0, 0, 0, 0, 0, 0, 0, 0, 0, 0, 0, 0, 0, 0, 0, 0, 0, 0, 0, 0, 0, 0, 0, 0, 0, 0, 0, 0, 0, 0, 0, 0, 0, 0, 0, 0, 0, 0, 0, 0, 0, 0, 0, 0, 0, 0, 0, 0, 0, 0, 0, 0, 0, 0, 0, 0, 0, 0, 0, 0, 0, 0, 0, 0, 0, 0, 0, 0, 0, 0, 0, 0, 0, 0, 0, 0, 0, 0, 0, 0, 0, 0, 0, 0, 0, 0, 0, 0, 0, 0, 0, 0, 0, 0, 0, 0, 0, 0, 0, 0, 0, 0, 0, 0, 0, 0, 0, 0, 0, 0, 0, 0, 0, 0, 0, 0, 0, 0, 0, 0, 0, 0, 0, 0, 0, 0, 0, 0, 0, 0, 0, 0, 0, 0, 0, 0, 0, 0, 0, 0, 0, 0, 0, 0, 0, 0, 0, 0, 0, 0, 0, 0, 0, 0, 0, 0, 0, 0, 0, 0, 0, 0, 0, 0, 0, 0, 0, 0, 0, 0, 0, 0, 0, 0, 0, 0, 0, 0, 0, 0, 0, 0, 0, 0, 0, 0, 0, 0, 0, 0, 0, 0, 0, 0, 0, 0, 0, 0, 0, 0, 0, 0, 0, 0, 0, 0, 0, 0, 0, 0, 0, 0, 0, 0, 0, 0, 0, 0, 0, 0, 0, 0, 0, 0, 0, 0, 0, 0, 0, 0, 0, 0, 0, 0, 0, 0, 0, 0, 0, 0, 0, 0, 0, 0, 0, 0, 0, 0, 0, 0, 0, 0, 0, 0, 0, 0, 0, 0, 0, 0, 0, 0, 0, 0, 0, 0, 0, 0, 0, 0, 0, 0, 0], "Size"=0, "IntnlStatus"=0, "IntnlErrCode"=93, "Alias16"=0, "Reserved"=0})   [LabVIEW 2016]
uses:
  Das16.llb/FromEng(array).VI
panel:
  out "Reserved":i32
  out "Alias16":u32
  out "IntnlErrCode":i32
  out "IntnlStatus":i32
  out "IntnlBoardNum":i32
  out "Size":i32
  out "32bit integer":i32
  out "Count":i32=2048
  out "?":i16[](graph)
  in  "AORange":i32(ring)=1 items=["Not Programmable"=0, "+- 20 V"=27, "+- 10 V"=1, "+- 5 V"=2, "+- 4 V"=28, "+- 2.5 V"=3, "+- 2 V"=29, "+- 1.67 V"=4, "+- 1.25 V"=5, "+- 1 V"=6, "+- .625 V"=7, "+- .5 V"=8, "+- .25 V"=30, "+- .2 V"=31, "+- .1 V"=9, "+- .05 V"=10, "+- .01 V"=11, "+- .005 V"=12, "0 - 10 V"=13, "0 - 5 V"=14, "0 - 4 V"=36, "0 - 2.5 V"=15, "0 - 2 V"=16, "0 - 1.67 V"=17, "0 - 1.25 V"=18, "0 - 1 V"=19, "0 - .5 V"=32, "0 - .25 V"=33, "0 - .2 V"=34, "0 - .1 V"=20, "0 - .02 V"=35, "0 - .01 V"=21, "4 - 20 mA"=22, "2 - 10 mA"=23, "1 - 5 mA"=24, ".5 - 2.5 mA"=25, "0 - 20 mA"=26]
  in  "ExtClock":bool
  in  "Simultaneous":bool=TRUE
  in  "Continuous":bool
  in  "InterChannel Delay":sgl=-1.0 format="%.2f"
  in  "Mode":i32(ring) items=["DEFAULTIO", "SINGLEIO", "DMAIO", "BLOCKIO", "BURSTIO"]
  in  "ExtTrigger":bool
  in  "Extclock":bool
  # "AInScBg.VI input parameters:"
  # "StopBg.VI output:"
  # "Output Buffer Paremeters"
  # "AOutScBb.VI Inputs"
  # "This example demonstrate simultaneous timed analog input and timed analog output functions on the same board.\nNote:\n    Not all hardware is supported by this function. Please refer to your hardware user manual for\n    more information"
  # "Options parameters (input to OptAIn.VI).\nDefault used for other option parameters."
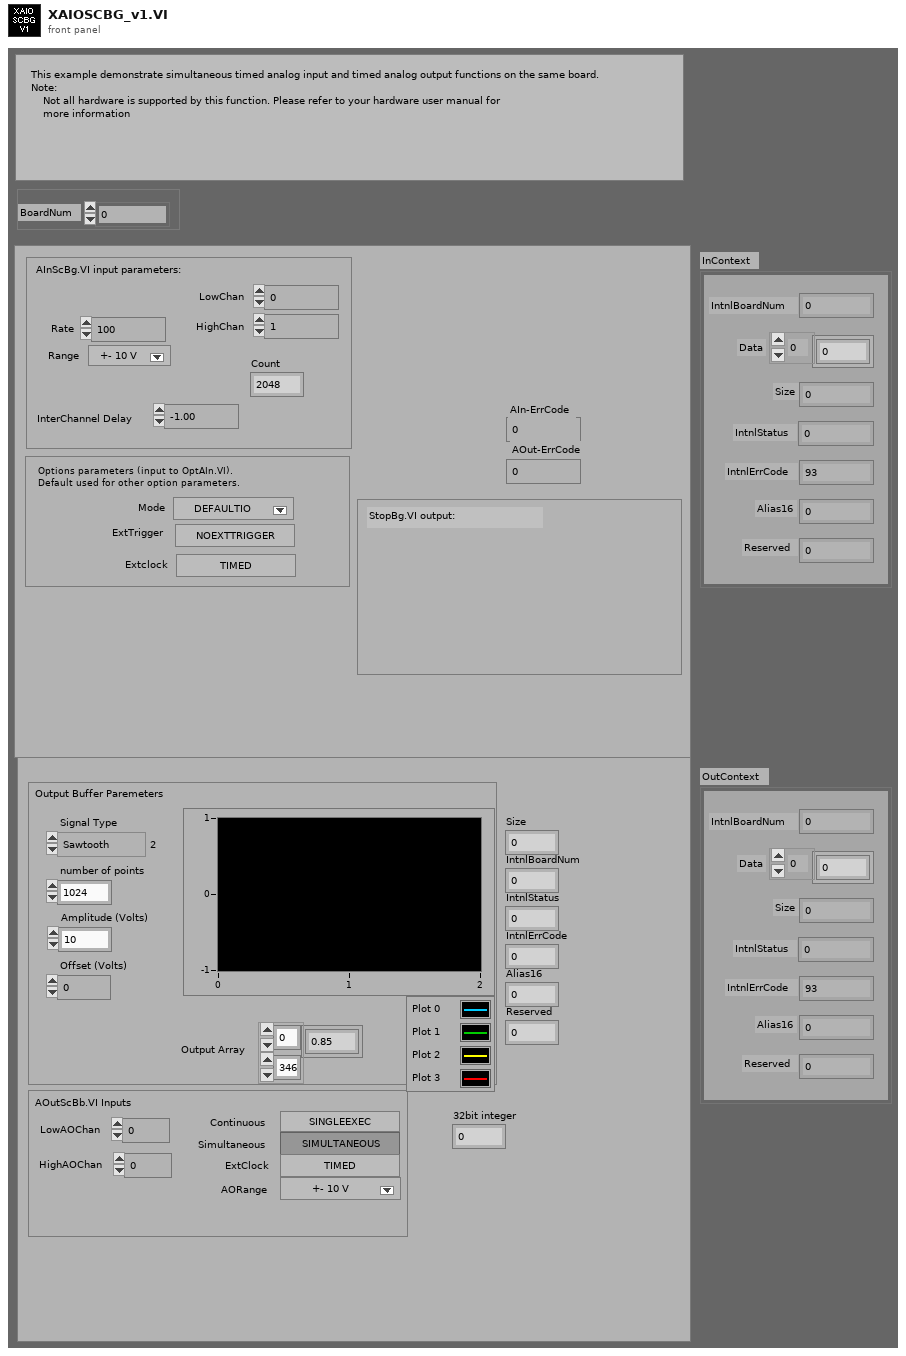
[diagram p1: front panel]
types:
  T1 = cluster{"IntnlBoardNum":i32, "Data":i16[], "Size":i32, "IntnlStatus":i32, "IntnlErrCode":i32, "Alias16":u32, "Reserved":i32}
  T2 = enum16{"Sine Wave", "Square Wave", "Sawtooth", "Triangle Wave"}
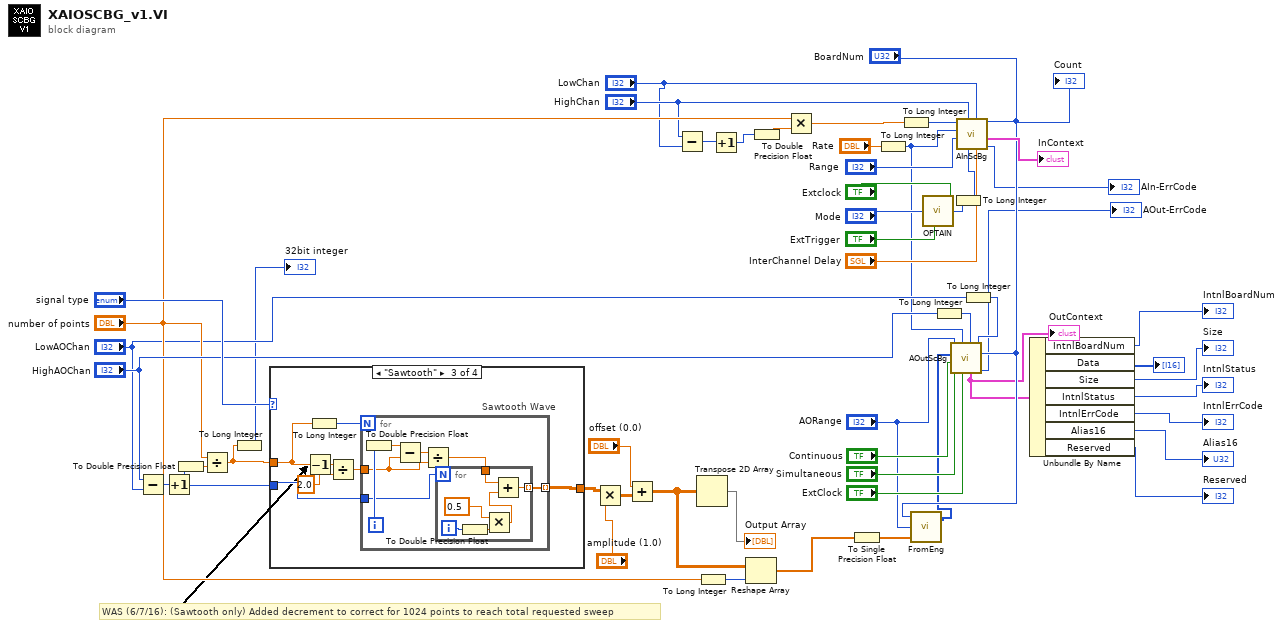
[diagram p0: block diagram]
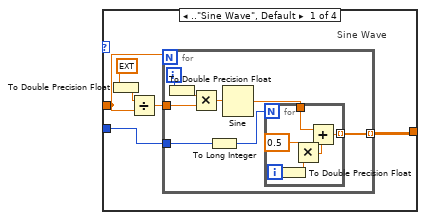
[diagram p2: hidden frame]
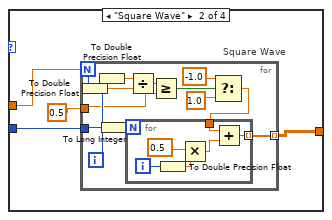
[diagram p3: hidden frame]
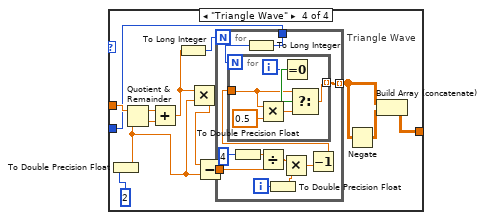
[diagram p4: hidden frame]
diagram:
  # "WAS (6/7/16): (Sawtooth only) Added decrement to correct for 1024 points to reach total requested sweep"
  n1 = Subtract(x="HighAOChan", y="LowAOChan") -> (x-y=w43:i32)
  n2 = Increment(x=w43) -> (x+1=w40:i32)
  n3 = To Double Precision Float(number=w40) -> (double precision float=w5:dbl)
  n4 = Divide(x="number of points", y=w5) -> (x/y=w1:dbl)
  n5 = To Long Integer(number=w1) -> (32bit integer=→"32bit integer":i32)
  n6 = case shown="\"Sawtooth\"" "signal type" {
    tunnel: w40 -> [w57 w76 w100 w123]
    tunnel: w1 -> [w56 w75 w101 w129]
    tunnel: [w54 w74 w98 w117] -> w11
    frame .."Sine Wave", Default {
      # "Sine Wave"
      n7 = To Double Precision Float(number=ext 6.283185307179586477) -> (double precision float=w55:dbl)
      n8 = Divide(x=w55, y=w56) -> (x/y=w58:dbl)
      n9 = for {
        N: w56 -> [_]
        tunnel: w58 -> [w65]
        tunnel: [w62] -> w54 mode=indexing
        tunnel: w57 -> [w64]
        i -> [w66]
        n10 = To Double Precision Float(number=w66) -> (double precision float=w60:dbl)
        n11 = Multiply(x=w60, y=w65) -> (x*y=w67:dbl)
        n12 = To Long Integer(number=w64) -> (32bit integer=w61:i32)
        n13 = Sine(x=w67) -> (sin(x)=w63:dbl)
        n14 = for {
          N: w61 -> [_]
          tunnel: w63 -> [w70]
          tunnel: [w69] -> w62 mode=indexing
          i -> [w72]
          n15 = To Double Precision Float(number=w72) -> (double precision float=w68:dbl)
          n16 = Multiply(x=0.5 ("Y offset between channels (0.5 V)"), y=w68) -> (x*y=w71:dbl)
          n17 = Add(x=w70, y=w71) -> (x+y=w69:dbl)
        }
      }
    }
    frame "Square Wave" {
      # "Square Wave"
      n18 = for {
        N: w75 -> [w82]
        tunnel: [w85] -> w74 mode=indexing
        tunnel: w76 -> [w84]
        tunnel: 0.5 -> [w83]
        i -> [w90]
        n19 = To Double Precision Float(number=w82) -> (double precision float=w79:dbl)
        n20 = To Double Precision Float(number=w90) -> (double precision float=w80:dbl)
        n21 = To Long Integer(number=w84) -> (32bit integer=w78:i32)
        n22 = Divide(x=w80, y=w79) -> (x/y=w89:dbl)
        n23 = Greater Or Equal?(x=w89, y=w83) -> (x >= y?=w86:bool)
        n24 = Select(t=-1.0, s=w86, f=1.0) -> (s? t:f=w81:dbl)
        n25 = for {
          N: w78 -> [_]
          tunnel: w81 -> [w93]
          tunnel: [w92] -> w85 mode=indexing
          i -> [w96]
          n26 = To Double Precision Float(number=w96) -> (double precision float=w91:dbl)
          n27 = Multiply(x=0.5 ("Y offset between channels (0.5 V)"), y=w91) -> (x*y=w94:dbl)
          n28 = Add(x=w93, y=w94) -> (x+y=w92:dbl)
        }
      }
    }
    frame "Sawtooth" {
      # "Sawtooth Wave"
      n29 = Decrement(x=w101) -> (x-1=w97:dbl)
      n30 = To Long Integer(number=w101) -> (32bit integer=w99:i32)
      n31 = Divide(x=w97, y=2.0) -> (x/y=w102:dbl)
      n32 = for {
        N: w99 -> [_]
        tunnel: w102 -> [w108]
        tunnel: [w107] -> w98 mode=indexing
        tunnel: w100 -> [w104]
        i -> [w109]
        n33 = To Double Precision Float(number=w109) -> (double precision float=w105:dbl)
        n34 = Subtract(x=w105, y=w108) -> (x-y=w110:dbl)
        n35 = Divide(x=w110, y=w108) -> (x/y=w106:dbl)
        n36 = for {
          N: w104 -> [_]
          tunnel: w106 -> [w113]
          tunnel: [w112] -> w107 mode=indexing
          i -> [w116]
          n37 = To Double Precision Float(number=w116) -> (double precision float=w111:dbl)
          n38 = Multiply(x=0.5 ("Y offset between channels (0.5 V)"), y=w111) -> (x*y=w114:dbl)
          n39 = Add(x=w113, y=w114) -> (x+y=w112:dbl)
        }
      }
    }
    frame "Triangle Wave" {
      # "Triangle Wave"
      n40 = To Double Precision Float(number=2) -> (double precision float=w119:dbl)
      n41 = Quotient & Remainder(x=w129, y=w119) -> (x-y*floor(x/y)=w121:dbl, floor(x/y)=w128:dbl)
      n42 = Add(x=w121, y=w128) -> (x+y=w127:dbl)
      n43 = To Long Integer(number=w127) -> (32bit integer=w118:i32)
      n44 = Multiply(x=w127, y=w119) -> (x*y=w124:dbl)
      n45 = Subtract(x=w124, y=w119) -> (x-y=w125:dbl)
      n46 = for {
        N: w118 -> [_]
        tunnel: w125 -> [w136]
        tunnel: w123 -> [w135]
        tunnel: [w133] -> w122 mode=indexing
        i -> [w139]
        n47 = To Double Precision Float(number=4 ("x")) -> (double precision float=w131:dbl)
        n48 = To Long Integer(number=w135) -> (32bit integer=w130:i32)
        n49 = Divide(x=w131, y=w136) -> (x/y=w138:dbl)
        n50 = To Double Precision Float(number=w139) -> (double precision float=w132:dbl)
        n51 = Multiply(x=w138, y=w132) -> (x*y=w137:dbl)
        n52 = Decrement(x=w137) -> (x-1=w134:dbl)
        n53 = for {
          N: w130 -> [_]
          tunnel: [w144] -> w133 mode=indexing
          tunnel: w134 -> [w143]
          i -> [w145]
          n54 = Multiply(x=w143, y=0.5) -> (x*y=w141:dbl)
          n55 = Equal To 0?(x=w145) -> (x = 0?=w146:bool)
          n56 = Select(t=w143, s=w146, f=w141) -> (s? t:f=w144:dbl)
        }
      }
      n57 = Negate(x=w122) -> (-x=w120:dbl[][])
      n58 = Build Array (concatenate)(w122, w120) -> (w117:dbl[][])
    }
  }
  n59 = Multiply(x=w11, y="amplitude (1.0)") -> (x*y=w37:dbl[][])
  n60 = Add(x="offset (0.0)", y=w37) -> (x+y=w35:dbl[][])
  n61 = Subtract(x="HighChan", y="LowChan") -> (x-y=w7:i32)
  n62 = Transpose 2D Array(2D array=w35) -> (transposed array=→"Output Array":dbl[][])
  n63 = To Long Integer(number="number of points") -> (32bit integer=w12:i32)
  n64 = Increment(x=w7) -> (x+1=w6:i32)
  n65 = Reshape Array(w35, w12) -> (w34:dbl[])
  n66 = To Double Precision Float(number=w6) -> (double precision float=w17:dbl)
  n67 = Multiply(x="number of points", y=w17) -> (x*y=w29:dbl)
  n68 = To Single Precision Float(number=w34) -> (single precision float=w10:sgl[])
  n69 = To Long Integer(number="Rate") -> (32bit integer=w16:i32)
  n70 = To Long Integer(number=w29) -> (32bit integer=w13:i32)
  "Count" <- w13
  n71 = call-poly "FromEng.VI"("EngUnits"=w10, "Range"="AORange", "BoardNum"="BoardNum") -> ("DA Data"=w27:u16[])  [unwired: 1 out]
  n72 = call "OPTAIN.VI"("Mode"="Mode", "ExtTrigger(false)"="ExtTrigger", "Extclock(false)"="Extclock") -> ("AInScanOptions"=w51:u32)  [unwired: 6 in]
  n73 = To Long Integer(number="HighAOChan") -> (32bit integer=w15:i32)
  n74 = To Long Integer(number=w51) -> (32bit integer=w4:i32)
  n75 = call "AInScBg.VI"("BoardNum"="BoardNum", "InterChannel Delay"="InterChannel Delay", "LowChan"="LowChan", "Options"=w4, "HighChan"="HighChan", "Range"="Range", "Rate"=w16, "Count"=w13) -> ("ErrCode"=→"AIn-ErrCode":i32, "Context"=→"InContext":T1)  [unwired: 1 in, 1 out]
  n76 = To Long Integer(number="LowAOChan") -> (32bit integer=w14:i32)
  n77 = call "AOutScBg.VI"("BoardNum"="BoardNum", "LowChan"=w14, "HighChan"=w15, "ExtClock"="ExtClock", "Rate"=w16, "Simultaneous"="Simultaneous", "Continuous"="Continuous", "DataArray"=w27, "Range"="AORange") -> ("ErrCode"=→"AOut-ErrCode":i32, "Context"=w26:T1)  [unwired: 1 out]
  "OutContext" <- w26
  n78 = Unbundle By Name(w26) -> ("IntnlBoardNum"=→"IntnlBoardNum":i32, "Data"=→"?":i16[], "Size"=→"Size":i32, "IntnlStatus"=→"IntnlStatus":i32, "IntnlErrCode"=→"IntnlErrCode":i32, "Alias16"=→"Alias16":u32, "Reserved"=→"Reserved":i32)
